vi "Launch Root Actor.vi"(8 "error in (no error)":errorcluster, 9 "Actor Name":string, 10 "Message Broker":refnum<class "Message Broker Interface.lvclass">, 11 "Mediated Asynchronous Actor in":refnum<class "Mediated Asynchronous Actor.lvclass">) -> (0 "error out":errorcluster, 3 "Command Actor Message Transport":refnum<class "Message Transport Interface.lvclass">)   [LabVIEW 2016, in "Stream Mediator.lvlib" / "Mediated Asynchronous Actor.lvclass"]
doc: "--\nCopyright © 2017 Composed SystemsI All rights reserved.\n\nAuthor: Jon McBee <jon.mcbee@composed.io>\n\nThis library is provided \"AS IS\" ,WITHOUT WARRANTIES OR\nCONDITIONS OF ANY KIND, either express or implied.\n\nComposed Systems -- composed.io\n\nStream 0.0.1.1\nJon McBee - Composed Systems\nCopyright (c) 2017, Composed Systems"
uses:
  <userlib>/Composed Systems/Stream/Mediator/Classes/Mediated Asynchronous Actor/Mediated Asynchronous Actor.lvclass
  <userlib>/Composed Systems/Stream/Mediator/Classes/Message Broker Interface/Message Broker Interface.lvclass
  <userlib>/Composed Systems/Stream/Mediator/Classes/Message Transport Interface/Message Transport Interface.lvclass
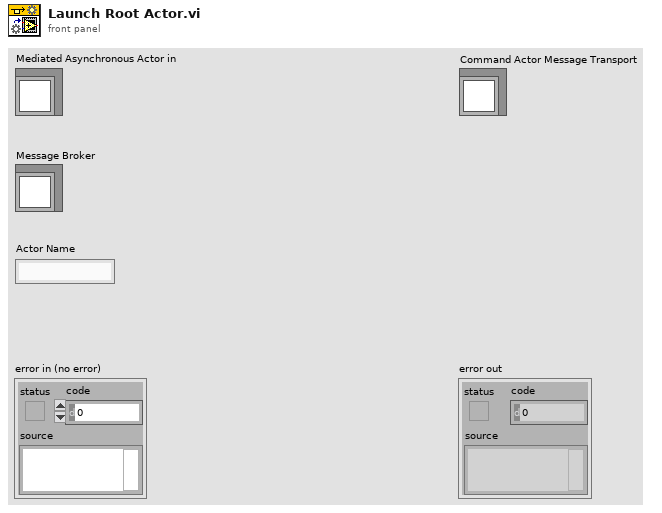
[diagram p1: front panel]
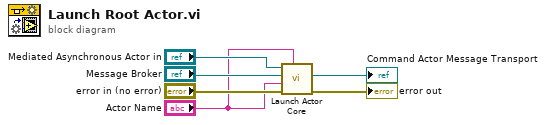
[diagram p0: block diagram]
diagram:
  n1 = call <userlib>:"Launch Actor Core.vi"("Host Name"="Actor Name", "error in (no error)"="error in (no error)", "Actor Name"="Actor Name", "Message Broker"="Message Broker", "Mediated Asynchronous Actor in"="Mediated Asynchronous Actor in") -> ("error out"=→"error out":errorcluster, "Message Transport"=→"Command Actor Message Transport":refnum<class "Message Transport Interface.lvclass">)  [unwired: 5 in]
